vi "Struct (Multi Type).vi"(6 "Typedef name":string, 7 "Typedef struct? (F)":bool, 8 "Struct name":string, 10 "Variables":cluster{"data type":string, "name":string}[](array[cluster]), 11 "String in":string) -> (3 "String out":string)   [LabVIEW 2013, in "C Header Generator.lvlib"]
uses:
  C Header Generator.lvlib
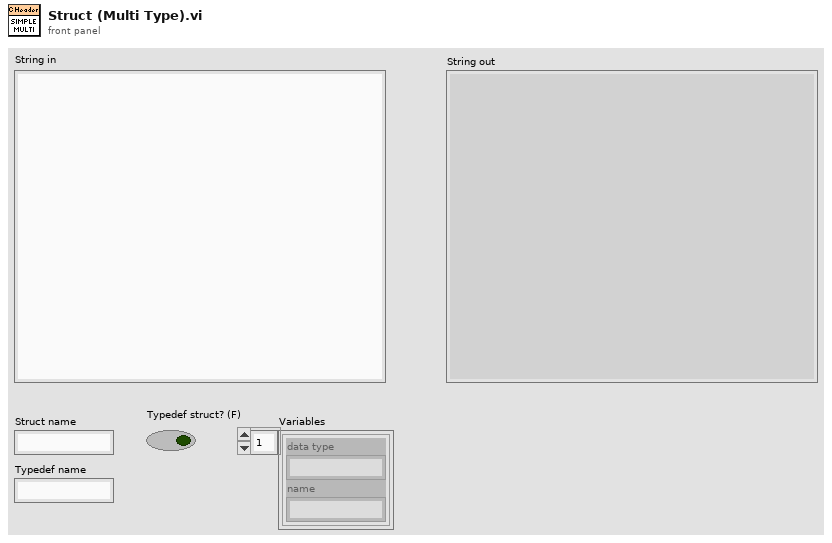
[diagram p1: front panel]
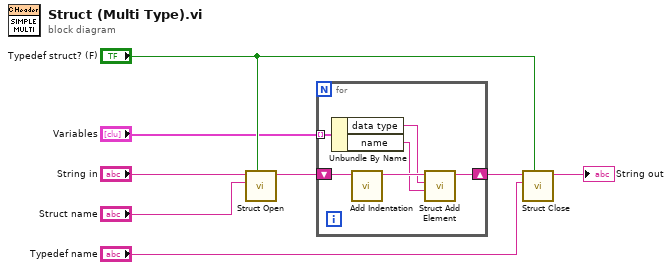
[diagram p0: block diagram]
diagram:
  n1 = call "Struct Open.vi"("Typedef struct? (F)"="Typedef struct? (F)", "Struct name"="Struct name", "String in"="String in") -> ("String out"=w6:string)  [unwired: 8 in]
  n2 = for {
    shift-right: [w14] -> w8
    shift-left: w6 -> [w13]
    tunnel: "Variables" -> [w11] mode=indexing
    n3 = Unbundle By Name(w11) -> ("data type"=w10:string, "name"=w9:string)
    n4 = call "Add Indentation.vi"("String in"=w13) -> ("String out"=w12:string)  [unwired: 10 in]
    n5 = call "Struct Add Element.vi"("Element name"=w9, "Element type"=w10, "String in"=w12) -> ("String out"=w14:string)  [unwired: 8 in]
  }
  n6 = call "Struct Close.vi"("Typedef struct? (F)"="Typedef struct? (F)", "Typedef name"="Typedef name", "String in"=w8) -> ("String out"=→"String out":string)  [unwired: 8 in]
